vi "TalonSRXVelocityToRPM.vi"(4 "Velocity (Raw Sensor Units per 100 ms)":i32) -> (1 "RPM":dbl)   [LabVIEW 2019]
panel:
  in  "constant":dbl=0.146484375 format="%#_13g"
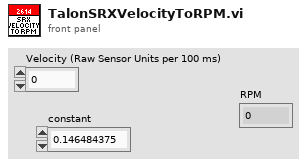
[diagram p1: front panel]
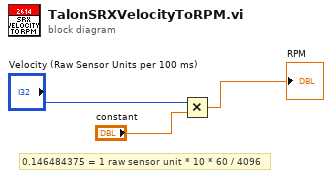
[diagram p0: block diagram]
diagram:
  # "0.146484375 = 1 raw sensor unit * 10 * 60 / 4096"
  n1 = Multiply(x="Velocity (Raw Sensor Units per 100 ms)", y="constant") -> (x*y=→"RPM":dbl)
